vi "Creator Queue.vi"(7 "jettl in":refnum<class "jettl.lvclass">, 8 "Priority?":bool, 9 "Msg Strategy":refnum<class "Msg Strategy.lvclass">, 10 "Queue Mailbox":refnum<data-value>) -> (5 "jettl out":refnum<class "jettl.lvclass">)   [LabVIEW 2021, in "jettl.lvlib" / "Addresses.lvlib"]
uses:
  Addresses.lvlib
  jettl/jettl.lvclass
  Msg Strategy/Msg Strategy.lvclass
  Addresses/Addresses.lvclass
  Self Queue/Self Queue.lvlib
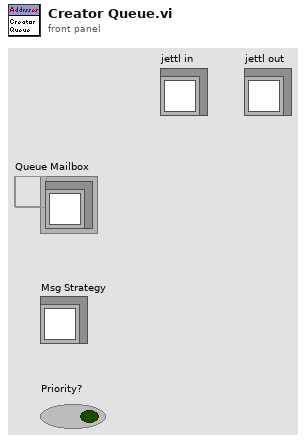
[diagram p1: front panel]
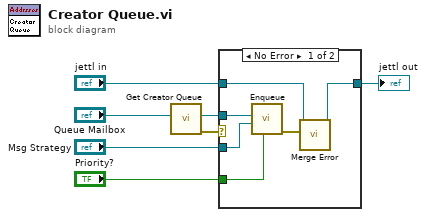
[diagram p0: block diagram]
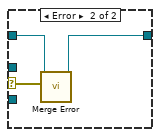
[diagram p2: hidden frame]
diagram:
  n1 = call "Get Creator Queue.vi"("Queue Mailbox"="Queue Mailbox") -> ("error out"=w1:errorcluster, "Creator Queue"=w5:refnum<data-value>)  [unwired: 9 in]
  n2 = case shown="No Error" w1 {
    selector: w1 -> [_ w14]
    tunnel: "Msg Strategy" -> [w12 _]
    tunnel: "Priority?" -> [w11 _]
    tunnel: w5 -> [w10 _]
    tunnel: "jettl in" -> [w9 w16]
    tunnel: [w8 w15] -> w2
    frame No Error {
      n3 = call "Enqueue.vi"("Priority?"=w11, "Msg Strategy"=w12, "Self Queue"=w10) -> ("error out"=w13:errorcluster)  [unwired: 8 in]
      n4 = call-dynamic "Merge Error.vi"("Error"=w13, "Merge Error in"=w9) -> ("Merge Error out"=w8:refnum<class "jettl.lvclass">)  [unwired: 9 in]
    }
    frame Error {
      n5 = call-dynamic "Merge Error.vi"("Error"=w14, "Merge Error in"=w16) -> ("Merge Error out"=w15:refnum<class "jettl.lvclass">)  [unwired: 9 in]
    }
  }
  "jettl out" <- w2
